vi "UTIL_Launch dynamic v1_0_0.vi"(5 "Sub Panel.Position":cluster{"Left":i32, "Top":i32}, 7 "General":string, 8 "error in (no error)":errorcluster, 10 "Array":string[](array[string]), 11 "Sub P ref":refnum<vi>) -> (0 "error out":errorcluster, 1 "String":string, 2 "queue out":refnum<queue>, 3 "Ref out":refnum<vi>)   [LabVIEW 2009]
doc: "UTIL_Launch dynamic v1_0_0.vi\n\nThis vi is used to dynamically launch another VI. This other VI can run in a subpanel or run stand alone in the background. \n\n1. = Path to VI \n2. = Wait until done (T/F)\n3. = In SubPanel (T/F)\n4. = Auto Disp. Ref\n5. = Overide Default open delay (3 sec.)\n6. = Variable 1\n7. = Variable 2\nCreated 2006 by:\n\nJ. Daren Suntych\nNational Analytics\n970-397-0764"
uses:
  <vilib>/addons/database/Connection.llb/Conn ObjectReference.ctl
  <vilib>/addons/database/NI_Database_API.lvlib
panel:
  in  "general 2":T2={"project directory"=path "C:/Documents and Settings/Owner/My Documents/AM/Projects/HRA/HRA_Suspension_Test_System", "User Name"="Chris Arabian", "User Level"="Chris Arabian", "valid login"=TRUE, "screen size"=1, "Screen Width"=1, "Screen Height"=1, "Login Password"="Chris Arabian", "Login User Name"="Chris Arabian", "DB Ref"=refnum, ".ini Resources"=[], "Control Refs"=[], "Error Ref out"=refnum}
  in  "Launch dynamic cluster":T3={"general"={"project directory"=path "C:/Documents and Settings/Owner/My Documents/AM/Projects/HRA/HRA_Suspension_Test_System", "User Name"="Chris Arabian", "User Level"="Chris Arabian", "valid login"=TRUE, "screen size"=1, "Screen Width"=1, "Screen Height"=1, "Login Password"="Chris Arabian", "Login User Name"="Chris Arabian", "DB Ref"=refnum, ".ini Resources"=[], "Control Refs"=[]}, "Path"="Chris Arabian", "Queue Name"="Chris Arabian", "Var. 1"="Chris Arabian", "Var. 2"="Chris Arabian", "Wait until Done"=TRUE, "Run in Subpanel"=TRUE, "Auto disp. Ref."=TRUE, "index of vi"=1, "Delay"="Chris Arabian", "sub queue name"="Chris Arabian", "vi reference"=refnum, "sub panel ref"=refnum}
  in  "Exit":bool
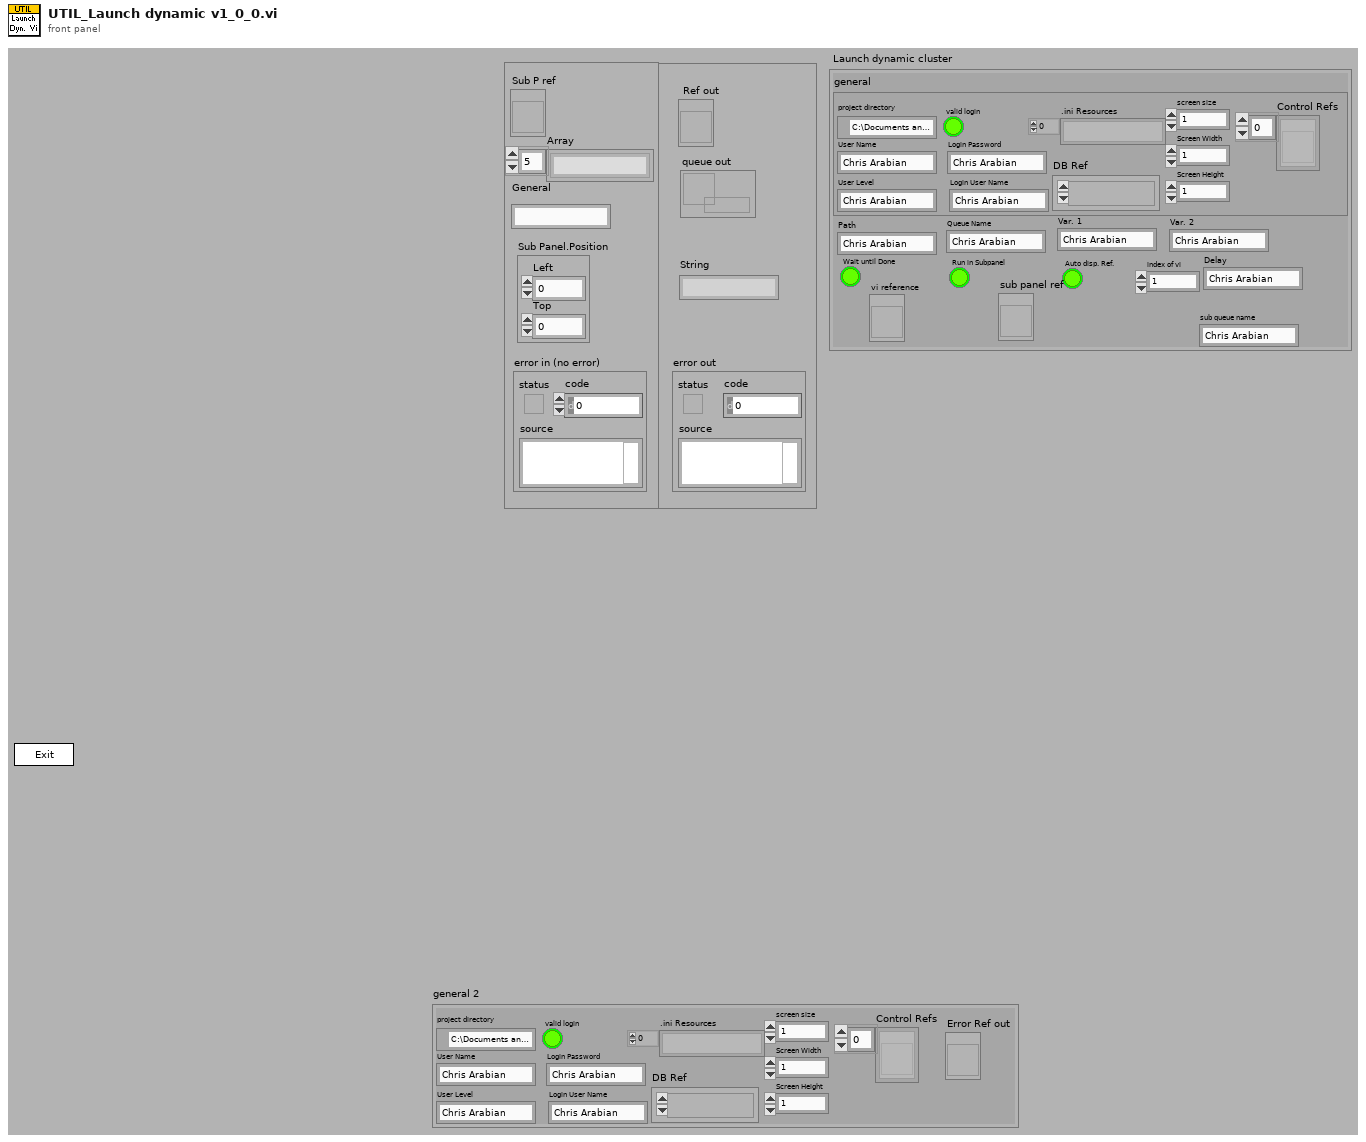
[diagram p1: front panel]
types:
  T1 = typedef "NI_Database_API.lvlib/Conn ObjectReference.ctl" = refnum<k1>
  T2 = cluster{"project directory":path, "User Name":string, "User Level":string, "valid login":bool, "screen size":i32, "Screen Width":i32, "Screen Height":i32, "Login Password":string, "Login User Name":string, "DB Ref":T1, ".ini Resources":string[], "Control Refs":refnum<vi>[], "Error Ref out":refnum<vi>}
  T3 = cluster{"general":cluster{"project directory":path, "User Name":string, "User Level":string, "valid login":bool, "screen size":i32, "Screen Width":i32, "Screen Height":i32, "Login Password":string, "Login User Name":string, "DB Ref":T1, ".ini Resources":string[], "Control Refs":refnum<vi>[]}, "Path":string, "Queue Name":string, "Var. 1":string, "Var. 2":string, "Wait until Done":bool, "Run in Subpanel":bool, "Auto disp. Ref.":bool, "index of vi":i32, "Delay":string, "sub queue name":string, "vi reference":refnum<vi>, "sub panel ref":refnum<vi>}
  T4 = enum32{"Bad", "Idle", "Run top level", "Running"}
  T5 = enum32{"Invalid", "Standard", "Closed", "Hidden", "Minimized", "Maximized"}
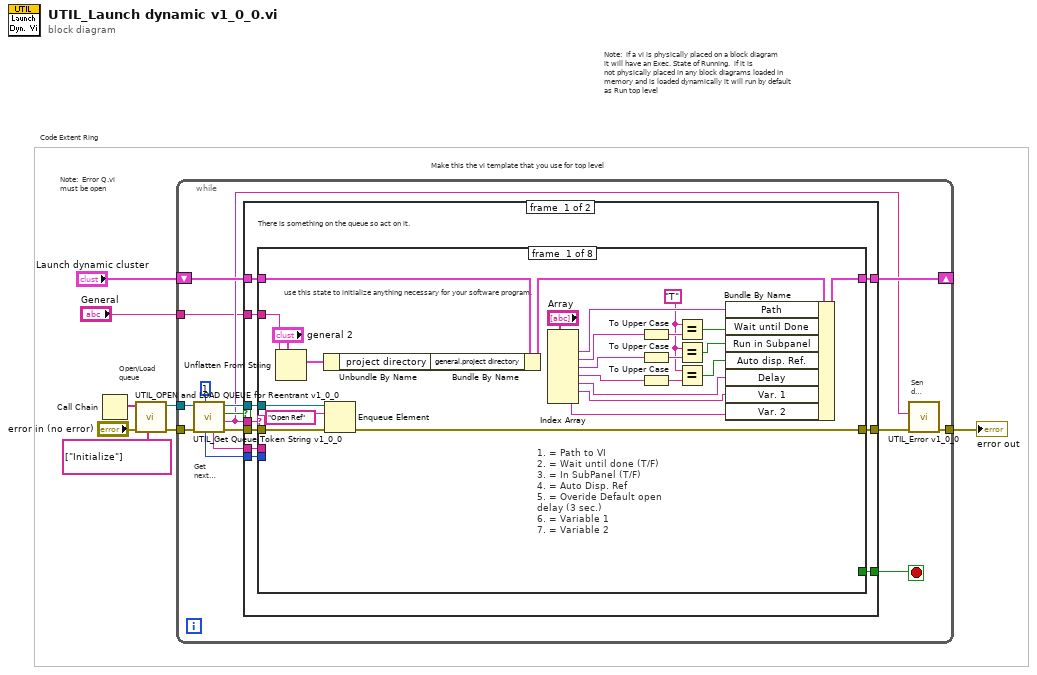
[diagram p0: block diagram]
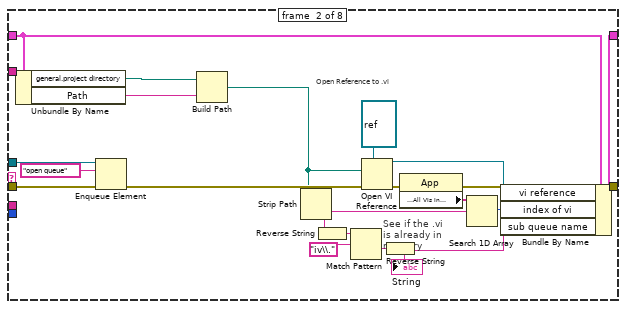
[diagram p2: hidden frame]
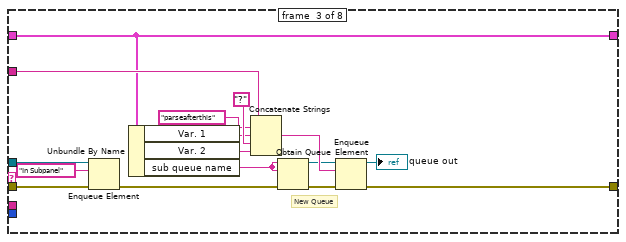
[diagram p3: hidden frame]
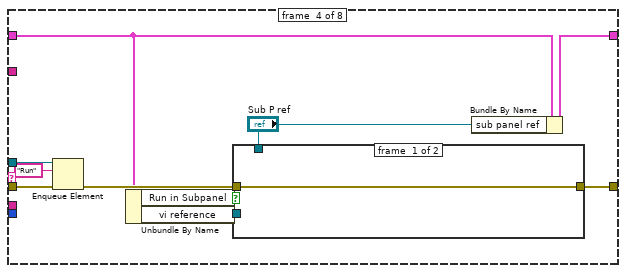
[diagram p4: hidden frame]
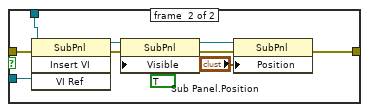
[diagram p5: hidden frame]
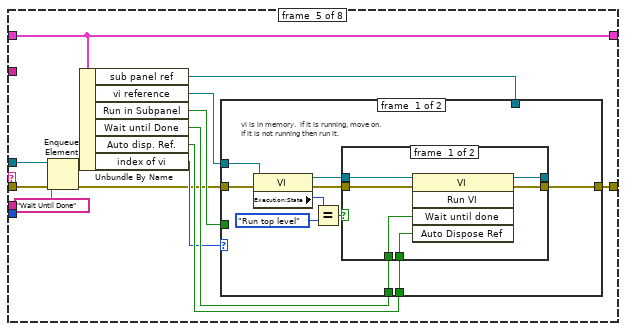
[diagram p6: hidden frame]
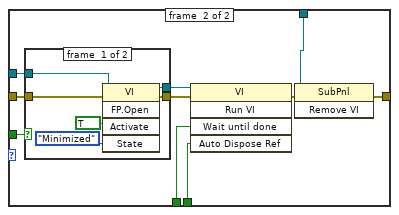
[diagram p8: hidden frame]
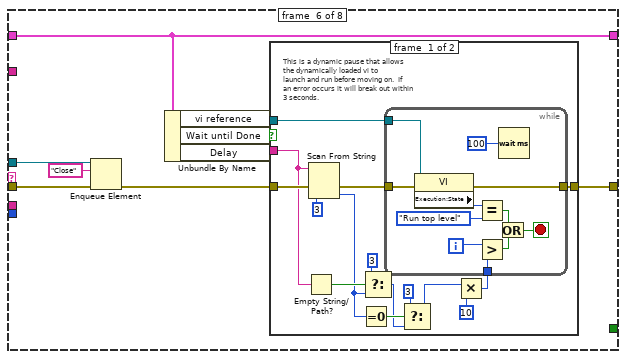
[diagram p10: hidden frame]
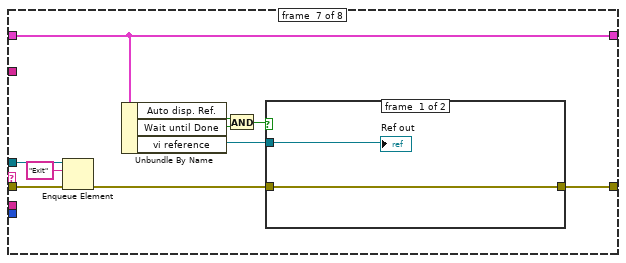
[diagram p12: hidden frame]
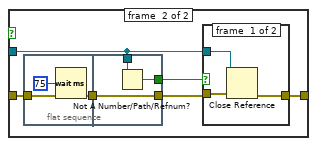
[diagram p13: hidden frame]
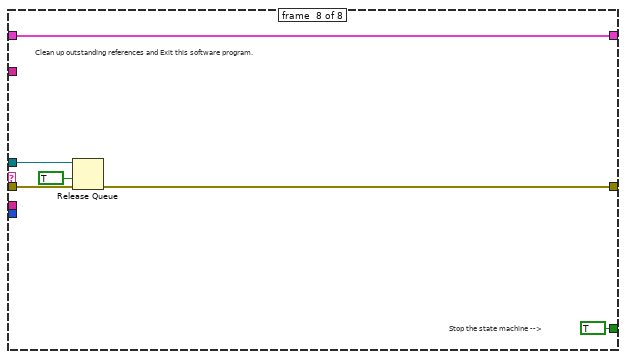
[diagram p15: hidden frame]
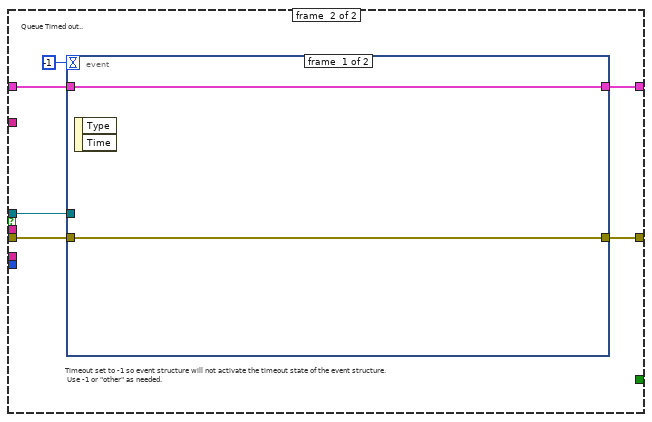
[diagram p16: hidden frame]
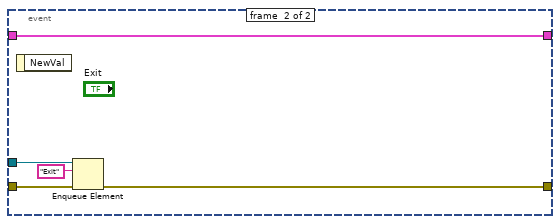
[diagram p17: hidden frame]
diagram:
  # "Note:  Error Q.vi\nmust be open"
  # "Open/Load\nqueue"
  # "Code Extent Ring"
  # "Make this the vi template that you use for top level"
  # "Note:  if a vi is physically placed on a block diagram\nit will have an Exec. State of Running.  if it is\nnot physically placed in any block diagrams loaded in\nmemory and is loaded dynamically it will run by default\nas Run top level"
  n1 = Call Chain() -> (call chain=w4:string[])
  n2 = call "UTIL_OPEN and LOAD QUEUE for Reentrant v1_0_0.vi"("Queue elements"=string[] ["Initialize"], "error in (no error)"="error in (no error)", "Call Chain"=w4) -> ("error out"=w2:errorcluster, "Queue out"=w5:refnum<queue>)  [unwired: 1 in, 6 out]
  n3 = while {
    tunnel: w5 -> [w16]
    tunnel: w2 -> [w17]
    shift-right: [w22] -> _
    shift-left: "Launch dynamic cluster" -> [w23]
    tunnel: [w19] -> w7
    tunnel: "General" -> [w9]
    stop <- w21 stop-if-true
    # "Get next\nstate"
    # "Send\nError"
    n4 = call "UTIL_Get Queue Token String v1_0_0.vi"("timeout in ms (-1)"=1, "error in (no error)"=w17, "queue"=w16) -> ("error out"=w18:errorcluster, "token string"=w10:string, "timed out?"=w11:bool, "queue out"=w12:refnum<queue>, "dup string"=w13:string, "offset past token"=w14:i32)  [unwired: 1 in, 2 out]
    n5 = case shown="True" w11 {
      tunnel: w12 -> [w32 w235]
      tunnel: w18 -> [w33 w237]
      tunnel: [w31 w236] -> w20
      tunnel: w23 -> [w29 w239]
      tunnel: [w30 w238] -> w22
      tunnel: [w28 _] -> w21
      tunnel: w13 -> [w26 _]
      tunnel: w14 -> [w27 _]
      tunnel: w10 -> [w25 _]
      tunnel: w9 -> [w24 _]
      frame #0 {
        # "There is something on the queue so act on it."
        n6 = case shown="\"Wait Until Done\"" w25 {
          tunnel: w33 -> [w59 w67 w86 w102 w120 w168 w209 w231]
          tunnel: w32 -> [w58 w68 w84 w103 w118 w166 w210 w230]
          tunnel: [w56 w73 w92 w105 w128 w173 w205 w228] -> w31
          tunnel: w29 -> [w35 w71 w80 w99 w125 w171 w207 w232]
          tunnel: [w55 w70 w80 w98 w125 w171 w207 w232] -> w30
          tunnel: [_ _ _ _ _ _ _ TRUE] -> w28
          tunnel: w27 -> [_ _ _ _ _ _ _ _]
          tunnel: w26 -> [_ _ _ _ _ _ _ _]
          tunnel: w24 -> [w36 _ w81 _ _ _ _ _]
          frame #0 {
            w44 = "T" ("x")
            # "1. = Path to VI \n2. = Wait until done (T/F)\n3. = In SubPanel (T/F)\n4. = Auto Disp. Ref\n5. = Overide Default open delay (3 sec.)\n6. = Variable 1\n7. = Variable 2"
            # "use this state to initialize anything necessary for your software program."
            n7 = Unflatten From String(type="general 2", binary string=w36) -> (value=w39:T2)  [unwired: 1 in, 4 out]
            n8 = Unbundle By Name(w39) -> ("project directory"=w38:path)
            n9 = Enqueue Element(queue=w58, element="Open Ref" ("queue element"), error in (no error)=w59) -> (error out=w56:errorcluster)  [unwired: 3 out]
            n10 = Bundle By Name(cluster=w35, "general.project directory"=w38) -> (w34:T3)
            n11 = Index Array(array="Array") -> (element #1=w54:string, element #2=w52:string, element #3=w48:string, element #4=w45:string, element #5=w43:string, element #6=w42:string, element #7=w40:string)  [unwired: 7 in]
            n12 = To Upper Case(1:w52) -> (0:w51:string)
            n13 = To Upper Case(1:w48) -> (0:w49:string)
            n14 = To Upper Case(1:w45) -> (0:w50:string)
            n15 = Equal?(x=w44, y=w51) -> (x = y?=w53:bool)
            n16 = Equal?(x=w44, y=w49) -> (x = y?=w47:bool)
            n17 = Equal?(x=w44, y=w50) -> (x = y?=w46:bool)
            n18 = Bundle By Name(cluster=w34, "Path"=w54, "Wait until Done"=w53, "Run in Subpanel"=w47, "Auto disp. Ref."=w46, "Delay"=w43, "Var. 1"=w42, "Var. 2"=w40) -> (w55:T3)
          }
          frame #1 {
            # "See if the .vi\nis already in memory"
            # "Open Reference to .vi"
            n19 = Unbundle By Name(w71) -> ("general.project directory"=w62:path, "Path"=w61:string)
            n20 = Enqueue Element(queue=w68, element="open queue", error in (no error)=w67) -> (error out=w66:errorcluster)  [unwired: 3 out]
            n21 = Build Path(base path=w62, name or relative path=w61) -> (appended path=w60:path)
            n22 = Strip Path(path=w60) -> (name=w72:string)  [unwired: 1 out]
            n23 = Reverse String(1:w72) -> (0:w78:string)
            n24 = Match Pattern(string=w78, regular expression="iv\\.") -> (after substring=w79:string)  [unwired: 4 out]
            n25 = Open VI Reference(type specifier VI Refnum (for type only)=refnum<vi> refnum, vi path=w60, error in (no error)=w66) -> (vi reference=w63:refnum<vi>, error out=w74:errorcluster)  [unwired: 3 out]
            n26 = Reverse String(1:w79) -> (0:w64:string)
            "String" <- w64
            n27 = property class="App"(error in=w74) -> (error out=w73:errorcluster, "Application:All VIs In Memory"=w75:string[])  [unwired: 1 in, 1 out]
            n28 = Search 1D Array(1D array=w75, element=w72) -> (index of element=w69:i32)  [unwired: 1 out]
            n29 = Bundle By Name(cluster=w71, "vi reference"=w63, "index of vi"=w69, "sub queue name"=w64) -> (w70:T3)
          }
          frame #2 {
            # "New Queue"
            n30 = Enqueue Element(queue=w84, element="In Subpanel", error in (no error)=w86) -> (error out=w85:errorcluster)  [unwired: 3 out]
            n31 = Unbundle By Name(w80) -> ("Var. 1"=w91:string, "Var. 2"=w90:string, "sub queue name"=w89:string)
            n32 = Concatenate Strings(w81, "parseafterthis" ("string"), w91, "?" ("string"), w90) -> (w95:string)
            n33 = Obtain Queue(name (unnamed)=w89, element data type=w89, error in (no error)=w85) -> (queue out=w88:refnum<queue>, error out=w87:errorcluster)  [unwired: 2 in, 1 out]
            n34 = Enqueue Element(queue=w88, element=w95, error in (no error)=w87) -> (queue out=→"queue out":refnum<queue>, error out=w92:errorcluster)  [unwired: 2 out]
          }
          frame #3 {
            n35 = Enqueue Element(queue=w103, element="Run", error in (no error)=w102) -> (error out=w101:errorcluster)  [unwired: 3 out]
            n36 = Unbundle By Name(w99) -> ("Run in Subpanel"=w104:bool, "vi reference"=w96:refnum<vi>)
            n37 = case shown="False" w104 {
              tunnel: w101 -> [w106 w116]
              tunnel: [w106 w110] -> w105
              tunnel: "Sub P ref" -> [_ w115]
              tunnel: w96 -> [_ w107]
              frame #0 {
              }
              frame #1 {
                n38 = invoke on="Invoke Node" class="SubPnl" method="Insert VI"(reference=w115, error in=w116, "VI Ref"=w107) -> (reference out=w114:refnum<vi>, error out=w113:errorcluster)  [unwired: 1 in, 2 out]
                n39 = property class="SubPnl"(reference=w114, error in=w113, "Visible"=TRUE) -> (reference out=w109:refnum<vi>, error out=w111:errorcluster)
                n40 = property class="SubPnl"(reference=w109, error in=w111, "Position"="Sub Panel.Position") -> (error out=w110:errorcluster)  [unwired: 1 out]
              }
            }
            n41 = Bundle By Name(cluster=w99, "sub panel ref"="Sub P ref") -> (w98:T3)
          }
          frame #4 {
            n42 = Enqueue Element(queue=w118, element="Wait Until Done", error in (no error)=w120) -> (error out=w119:errorcluster)  [unwired: 3 out]
            n43 = Unbundle By Name(w125) -> ("sub panel ref"=w124:refnum<vi>, "vi reference"=w127:refnum<vi>, "Run in Subpanel"=w126:bool, "Wait until Done"=w123:bool, "Auto disp. Ref."=w122:bool, "index of vi"=w121:i32)
            n44 = case shown="-1" w121 {
              tunnel: w119 -> [w137 w156]
              tunnel: [w138 w148] -> w128
              tunnel: w127 -> [w131 w153]
              tunnel: w123 -> [w130 w150]
              tunnel: w122 -> [w129 w152]
              tunnel: w126 -> [_ w151]
              tunnel: w124 -> [_ w147]
              frame #0 {
                # "vi is in memory.  if it is running, move on.\nIf it is not running then run it."
                n45 = property class="VI"(reference=w131, error in=w137) -> (reference out=w135:refnum<vi>, error out=w136:errorcluster, "Execution:State"=w134:T4)
                n46 = Equal?(x=w134, y=T4."Run top level") -> (x = y?=w132:bool)
                n47 = case shown="False" w132 {
                  tunnel: [w144 w145] -> w138
                  tunnel: [w143 w146] -> _
                  tunnel: w136 -> [w142 w145]
                  tunnel: w135 -> [w141 w146]
                  tunnel: w130 -> [w139 _]
                  tunnel: w129 -> [w140 _]
                  frame #0 {
                    n48 = invoke class="VI" method="Run VI"(reference=w141, error in=w142, "Wait until done"=w139, "Auto Dispose Ref"=w140) -> (reference out=w143:refnum<vi>, error out=w144:errorcluster)  [unwired: 1 in, 3 out]
                  }
                  frame #1 {
                  }
                }
              }
              frame #1 {
                n49 = case shown="False" w151 {
                  tunnel: w156 -> [w162 w163]
                  tunnel: [w159 w164] -> w155
                  tunnel: [w158 w163] -> w154
                  tunnel: w153 -> [w157 w164]
                  frame #0 {
                    n50 = invoke class="VI" method="FP.Open"(reference=w157, error in=w162, "Activate"=TRUE, "State"=T5."Minimized") -> (reference out=w159:refnum<vi>, error out=w158:errorcluster)  [unwired: 1 in, 3 out]
                  }
                  frame #1 {
                  }
                }
                n51 = invoke class="VI" method="Run VI"(reference=w155, error in=w154, "Wait until done"=w150, "Auto Dispose Ref"=w152) -> (error out=w149:errorcluster)  [unwired: 1 in, 4 out]
                n52 = invoke class="SubPnl" method="Remove VI"(reference=w147, error in=w149) -> (error out=w148:errorcluster)  [unwired: 1 in, 2 out]
              }
            }
          }
          frame #5 {
            n53 = Enqueue Element(queue=w166, element="Close", error in (no error)=w168) -> (error out=w167:errorcluster)  [unwired: 3 out]
            n54 = Unbundle By Name(w171) -> ("vi reference"=w172:refnum<vi>, "Wait until Done"=w170:bool, "Delay"=w169:string)
            n55 = case shown="False" w170 {
              tunnel: [w188 w200] -> w173
              tunnel: w172 -> [w187 _]
              tunnel: w167 -> [w180 w200]
              tunnel: w169 -> [w174 _]
              frame #0 {
                # "This is a dynamic pause that allows\nthe dynamically loaded vi to \nlaunch and run before moving on.  If \nan error occurs it will break out within\n3 seconds."
                n56 = Empty String/Path?(string/path=w174) -> (empty?=w184:bool)
                n57 = Scan From String(input string=w174, error in=w180, default 1=3 ("Delay to Start (s)")) -> (error out=w181:errorcluster, output 1=w177:i32)  [unwired: 2 in, 2 out]
                n58 = Equal To 0?(x=w177) -> (x = 0?=w178:bool)
                n59 = Select(t=3 ("Delay to Start (s)"), s=w184, f=w177) -> (s? t:f=w176:i32)
                n60 = Select(t=3 ("Delay to Start (s)"), s=w178, f=w176) -> (s? t:f=w179:i32)
                n61 = Multiply(x=w179, y=10) -> (x*y=w185:i32)
                n62 = while {
                  tunnel: w187 -> [w199]
                  tunnel: w181 -> [w198]
                  tunnel: [w191] -> w188
                  tunnel: w185 -> [w189]
                  i -> [w195]
                  stop <- w192 stop-if-true
                  n63 = property class="VI"(reference=w199, error in=w198) -> (error out=w191:errorcluster, "Execution:State"=w197:T4)  [unwired: 1 out]
                  n64 = Equal?(x=w197, y=T4."Run top level" ("Execution:State")) -> (x = y?=w194:bool)
                  n65 = Greater?(x=w195, y=w189) -> (0:w193:bool)
                  n66 = Or(x=w194, y=w193) -> (x .or. y?=w192:bool)
                  n67 = Wait (ms)(milliseconds to wait=u32 100) -> ()  [unwired: 1 out]
                }
              }
              frame #1 {
              }
            }
          }
          frame #6 {
            n68 = Enqueue Element(queue=w210, element="Exit", error in (no error)=w209) -> (error out=w206:errorcluster)  [unwired: 3 out]
            n69 = Unbundle By Name(w207) -> ("Auto disp. Ref."=w203:bool, "Wait until Done"=w204:bool, "vi reference"=w201:refnum<vi>)
            n70 = And(x=w203, y=w204) -> (x .and. y?=w202:bool)
            n71 = case shown="True" w202 {
              tunnel: w206 -> [w212 w217]
              tunnel: [w212 w218] -> w205
              tunnel: w201 -> [w211 w215]
              frame #0 {
                "Ref out" <- w211
              }
              frame #1 {
                n72 = flat-sequence {
                  tunnel: w217 -> [w219]
                  tunnel: [w219] -> w216
                  tunnel: [w223] -> w213
                  tunnel: w216 -> [w223]
                  tunnel: w215 -> [w222]
                  tunnel: [w221] -> w214
                  frame #0 {
                    n73 = Wait (ms)(milliseconds to wait=u32 75) -> ()  [unwired: 1 out]
                  }
                  frame #1 {
                    n74 = Not A Number/Path/Refnum?(number/path/refnum=w222) -> (NaN/Path/Refnum?=w221:bool)
                  }
                }
                n75 = case shown="True" w214 {
                  tunnel: w215 -> [w226 _]
                  tunnel: w213 -> [w225 w227]
                  tunnel: [w224 w227] -> w218
                  frame #0 {
                    n76 = Close Reference(reference=w226, error in (no error)=w225) -> (error out=w224:errorcluster)
                  }
                  frame #1 {
                  }
                }
              }
            }
          }
          frame #7 {
            # "Stop the state machine -->"
            # "Clean up outstanding references and Exit this software program."
            n77 = Release Queue(queue=w230, force destroy? (F)=TRUE, error in (no error)=w231) -> (error out=w228:errorcluster)  [unwired: 2 out]
          }
        }
      }
      frame #1 {
        # "Timeout set to -1 so event structure will not activate the timeout state of the event structure.\n Use -1 or \"other\" as needed."
        # "Queue Timed out.."
        n78 = event shown="[1] \"Exit\": Value Change" {
          selector: _ -> [_ _]
          dyn-events: _ -> [_ _]
          timeout: -1 -> [_ _]
          tunnel: [w241 w246] -> w238
          tunnel: w239 -> [w241 w246]
          tunnel: [w240 w243] -> w236
          tunnel: w237 -> [w240 w244]
          tunnel: w235 -> [_ w245]
          event #0 {
            n79 = event-data() -> ()  [unwired: 3 out]
          }
          event #1 {
            n80 = event-data() -> ()  [unwired: 2 out]
            n81 = Enqueue Element(queue=w245, element="Exit", error in (no error)=w244) -> (error out=w243:errorcluster)  [unwired: 3 out]
          }
        }
      }
    }
    n82 = call "UTIL_Error v1_0_0.vi"("error in (no error)"=w20, "State"=w10) -> ("error out"=w19:errorcluster)  [unwired: 1 in, 8 out]
  }
  "error out" <- w7
